vi "Read reconn_timeout.vi"(8 "error in (no error)":errorcluster, 11 "Master CR in":refnum<class "WebSocket Client CR.lvclass">) -> (0 "error out":errorcluster, 2 "reconn_timeout":i32=3000 min=10 max=240000 step=1, 3 "Master CR out":refnum<class "WebSocket Client CR.lvclass">)   [LabVIEW 2021, in "WebSockets.lvlib" / "WebSocket Client CR.lvclass"]
uses:
  WebSocket Client CR.lvclass
  WebSocket Client CR.lvclass/WebSocket Client CR.ctl
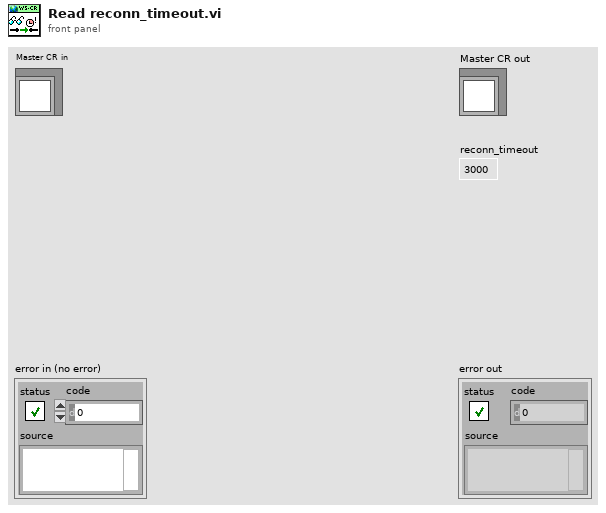
[diagram p1: front panel]
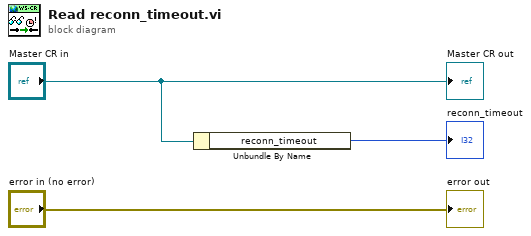
[diagram p0: block diagram]
diagram:
  n1 = Unbundle By Name("Master CR in") -> ("reconn_timeout"=→"reconn_timeout":i32)
  "error out" <- "error in (no error)"
  "Master CR out" <- "Master CR in"
